vi "5vote.vi"(10 "Input":bool=TRUE) -> (2 "vote5":bool)   [LabVIEW 2016, in "KevLib01.lvlib"]
uses:
  KevLib01.lvlib
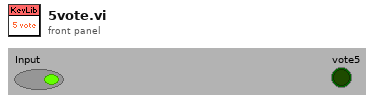
[diagram p1: front panel]
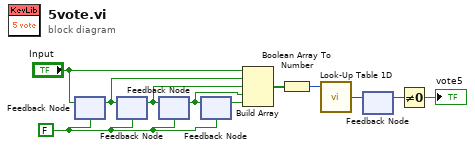
[diagram p0: block diagram]
diagram:
  w3 = FALSE ("Input")
  n1 = feedback-in #1("Input") -> ()
  n2 = feedback #1(w3) -> (w10:bool)
  n3 = feedback-in #2(w10) -> ()
  n4 = feedback #2(w3) -> (w9:bool)
  n5 = feedback-in #3(w9) -> ()
  n6 = feedback #3(w3) -> (w8:bool)
  n7 = feedback-in #4(w8) -> ()
  n8 = feedback #4(w3) -> (w7:bool)
  n9 = Build Array("Input", w10, w9, w8, w7) -> (w6:bool[])
  n10 = Boolean Array To Number(Boolean array=w6) -> (number=w5:u8)
  n11 = call "Look-Up Table 1D"("address"=w5) -> ("data out"=w2:u8)  [unwired: 8 in]
  n12 = feedback-in #5(w2) -> ()
  n13 = feedback #5() -> (w1:u8)  [unwired: 1 out]
  n14 = Not Equal To 0?(x=w1) -> (x != 0?=→"vote5":bool)
